vi "Global 2.vi"() -> ()   [LabVIEW 2019]
panel:
  out "Horizontal Angle":dbl
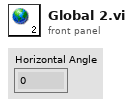
[diagram p1: front panel]
diagram:
